vi "clamp.vi"(1 "Min":dbl, 2 "Input":dbl, 3 "Max":dbl) -> (0 "Output":dbl)   [LabVIEW 2014]
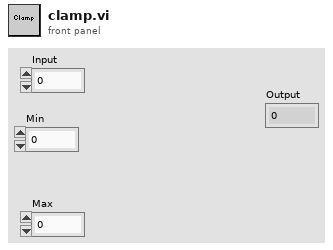
[diagram p1: front panel]
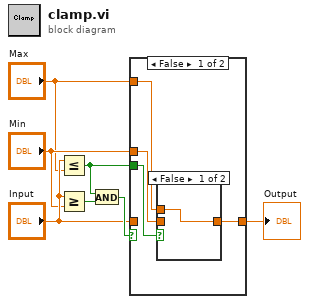
[diagram p0: block diagram]
diagram:
  n1 = Less Or Equal?(x="Input", y="Max") -> (x <= y?=w3:bool)
  n2 = Greater Or Equal?(x="Input", y="Min") -> (x >= y?=w7:bool)
  n3 = And(x=w3, y=w7) -> (x .and. y?=w6:bool)
  n4 = case shown="False" w6 {
    tunnel: "Input" -> [_ w14]
    tunnel: [w9 w14] -> w4
    tunnel: w3 -> [w11 _]
    tunnel: "Min" -> [w10 _]
    tunnel: "Max" -> [w8 _]
    frame False {
      n5 = case shown="False" w11 {
        tunnel: w10 -> [_ w13]
        tunnel: [w12 w13] -> w9
        tunnel: w8 -> [w12 _]
        frame False {
        }
        frame True {
        }
      }
    }
    frame True {
    }
  }
  "Output" <- w4
